vi "Initialize.vi"(8 "error in (no error)":errorcluster, 11 "WeatherStation in":refnum<class "WeatherStation.lvclass">) -> (0 "error out":errorcluster, 3 "WeatherStation out":refnum<class "WeatherStation.lvclass">)   [LabVIEW 2018, in "WeatherStation.lvclass"]
uses:
  WeatherStation.lvclass
  Server/Server.lvclass
  Comm/Stream/Stream.lvclass
  Log/Log.lvclass
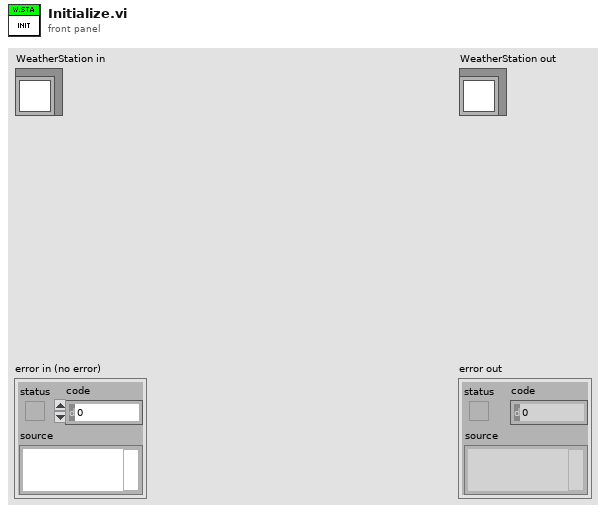
[diagram p1: front panel]
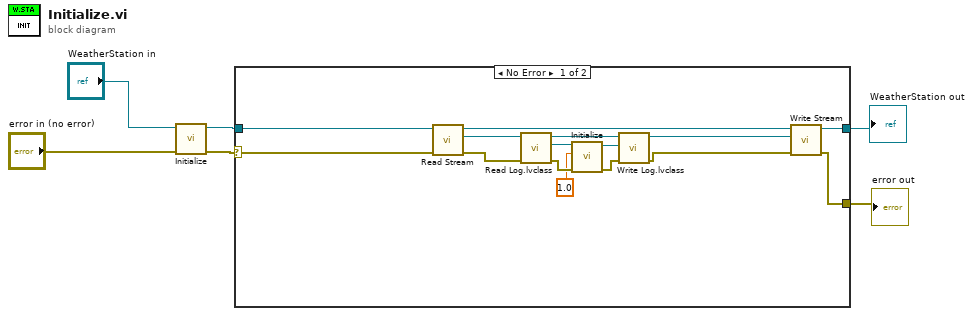
[diagram p0: block diagram]
diagram:
  n1 = call-parent "Initialize.vi"("error in (no error)"="error in (no error)", "Server in"="WeatherStation in") -> ("error out"=w3:errorcluster, "Server out"=w4:refnum<class "WeatherStation.lvclass">)  [unwired: 8 in]
  n2 = case shown="No Error" w3 {
    selector: w3 -> [w9 w22]
    tunnel: w4 -> [w10 w23]
    tunnel: [w20 w23] -> w2
    tunnel: [w19 w22] -> w1
    frame No Error {
      n3 = call-dynamic "Read Stream.vi"("error in (no error)"=w9, "Server in"=w10) -> ("error out"=w7:errorcluster, "Stream.lvclass"=w8:refnum<class "Stream.lvclass">, "Server out"=w21:refnum<class "WeatherStation.lvclass">)  [unwired: 7 in]
      n4 = call-dynamic "Read Log.lvclass.vi"("error in (no error)"=w7, "Comm in"=w8) -> ("error out"=w15:errorcluster, "Log.lvclass"=w17:refnum<class "Log.lvclass">, "Comm out"=w18:refnum<class "Stream.lvclass">)  [unwired: 7 in]
      n5 = call-dynamic "Initialize.vi"("error in (no error)"=w15, "Level"=1.0, "Log in"=w17) -> ("error out"=w14:errorcluster, "Log out"=w16:refnum<class "Log.lvclass">)  [unwired: 7 in]
      n6 = call-dynamic "Write Log.lvclass.vi"("error in (no error)"=w14, "Log.lvclass"=w16, "Comm in"=w18) -> ("error out"=w12:errorcluster, "Comm out"=w13:refnum<class "Stream.lvclass">)  [unwired: 7 in]
      n7 = call-dynamic "Write Stream.vi"("error in (no error)"=w12, "Stream.lvclass"=w13, "Server in"=w21) -> ("error out"=w19:errorcluster, "Server out"=w20:refnum<class "WeatherStation.lvclass">)  [unwired: 7 in]
    }
    frame Error {
    }
  }
  "error out" <- w1
  "WeatherStation out" <- w2
